vi "Load_Mode.vi"() -> ()   [LabVIEW 2016]
panel:
  in  "Load Mode":bool
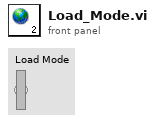
[diagram p1: front panel]
diagram:
